vi "http check to keep listening.vi"(11 "application request in":T1) -> (2 "stop listening":bool, 3 "application request out":T1)   [LabVIEW 2013]
uses:
  http request.ctl
  http method.ctl
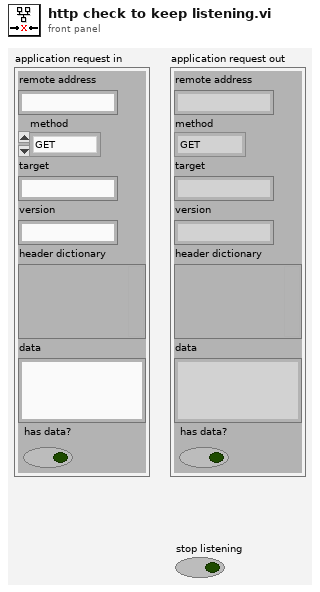
[diagram p1: front panel]
types:
  T1 = typedef "http request.ctl" = cluster{"remote address":string, "method":T2, "target":string, "version":string, "header dictionary":variant, "data":string, "has data?":bool}
  T2 = typedef "http method.ctl" = enum16{"GET", "POST", "PUT", "DELETE", "HEAD", "OPTIONS", "upgrade"}
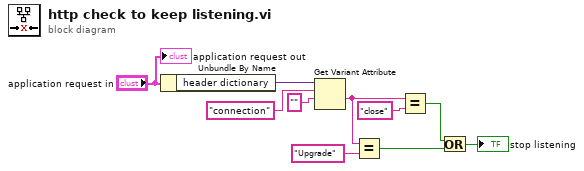
[diagram p0: block diagram]
diagram:
  n1 = Unbundle By Name("application request in") -> ("header dictionary"=w9:variant)
  n2 = Get Variant Attribute(Variant=w9, name="connection", default value (empty Variant)="" ("name")) -> (value=w1:string)  [unwired: 1 in, 3 out]
  n3 = Equal?(x=w1, y="Upgrade" ("name")) -> (x = y?=w5:bool)
  n4 = Equal?(x=w1, y="close" ("name")) -> (x = y?=w3:bool)
  n5 = Or(x=w3, y=w5) -> (x .or. y?=→"stop listening":bool)
  "application request out" <- "application request in"
